vi "log analysis_gps.vi"() -> ()   [LabVIEW 2019] (continued)
0 0\trobot status\t323.592230\t41.689812\t11.246000\t-1.200662\t-1.937489\t150.317707\t0.261000\t0.044000\n\t\n15:30:30.4\tlog_raw\tgps_raw\t\tsystem status\tnormal 2 28.000000 0 0\trobot status\t323.484203\t41.766278\t11.242100\t-1.080469\t-2.157866\t150.215109\t0.275000\t0.023000\n\t\n15:30:30.9\tlog_raw\tgps_raw\t\tsystem status\tnormal 2 28.000000 0 0\trobot status\t323.368044\t41.849297\t11.238300\t-0.983089\t-2.252578\t150.171279\t0.264000\t0.055000\n\t\n15:30:31.4\tlog_raw\tgps_raw\t\tsystem status\tnormal 2 28.000000 0 0\trobot status\t323.251094\t41.933868\t11.233500\t-0.837664\t-2.448431\t150.085808\t0.287000\t0.017000\n\t\n15:30:31.9\tlog_raw\tgps_raw\t#INSPVAXA,USB3,0,50.0,FINESTEERING,2107,282649.900,02000000,471d,15824;INS_ALIGNMENT_COMPLETE,INS_RTKFIXED,37.37050893925,126.72448297158,11.2267,22.3000,0.1903,-0.2023,-0.0241,-0.768669991,-2.369260824,300.015949522,0.4461,0.2933,0.5487,0.1140,0.0923,0.0771,0.0990,0.1039,4.8348,0f000001,0*dea76ac5\n\tsystem status\tnormal 2 28.000000 0 0\trobot status\t323.122038\t42.028367\t11.226700\t-0.768670\t-2.369261\t149.984050\t0.259000\t0.049000\n\t\n15:30:32.4\tlog_raw\tgps_raw\t#INSPVAXA,USB3,0,51.5,FINESTEERING,2107,282650.400,02000000,471d,15824;INS_ALIGNMENT_COMPLETE,INS_RTKFIXED,37.37050972480,126.72448163294,11.2213,22.3000,0.2048,-0.2320,-0.0314,-0.685414349,-2.106294081,300.095837477,0.4453,0.2931,0.5488,0.1140,0.0923,0.0771,0.0990,0.1038,4.8348,0f000001,0*243c57b4\n\tsystem status\tnormal 2 28.000000 0 0\trobot status\t323.003463\t42.115555\t11.221300\t-0.685414\t-2.106294\t149.904163\t0.308000\t-0.015000\n\t\n15:30:32.9\tlog_raw\tgps_raw\t\tsystem status\tnormal 2 28.000000 0 0\trobot status\t322.902785\t42.190545\t11.217300\t-0.695969\t-2.083132\t149.879193\t0.320000\t-0.056000\n\t\n15:30:33.4\tlog_raw\tgps_raw\t\tsystem status\tnormal 2 28.000000 0 0\trobot status\t322.782651\t42.278318\t11.212600\t-0.741534\t-2.009396\t149.782381\t0.332000\t-0.058000\n\t\n15:30:33.9\tlog_raw\tgps_raw\t#INSPVAXA,USB3,0,45.5,FINESTEERING,2107,282651.900,02000000,471d,15824;INS_ALIGNMENT_COMPLETE,INS_RTKFIXED,37.37051201880,126.72447778068,11.2078,22.3000,0.1916,-0.2205,-0.0248,-0.576530745,-1.861777705,300.300269268,0.4449,0.2931,0.5488,0.1139,0.0923,0.0771,0.0990,0.1038,4.8347,0f000001,0*af26017a\n\tsystem status\tnormal 2 28.000000 0 0\trobot status\t322.662236\t42.370167\t11.207800\t-0.576531\t-1.861778\t149.699731\t0.299000\t-0.003000\n\t\n15:30:34.4\tlog_raw\tgps_raw\t\tsystem status\tnormal 2 28.000000 0 0\trobot status\t322.556126\t42.447985\t11.205500\t-0.579348\t-1.879669\t149.599843\t0.304000\t-0.005000\n\t\n15:30:34.9\tlog_raw\tgps_raw\t\tsystem status\tnormal 2 28.000000 0 0\trobot status\t322.440446\t42.533452\t11.202500\t-0.656280\t-1.866283\t149.472784\t0.304000\t-0.004000\n\t\n15:30:35.4\tlog_raw\tgps_raw\t\tsystem status\tnormal 2 28.000000 0 0\trobot status\t322.324996\t42.617118\t11.198800\t-0.815807\t-1.929924\t149.361970\t0.259000\t0.044000\n\t\n15:30:35.9\tlog_raw\tgps_raw\t#INSPVAXA,USB3,0,51.5,FINESTEERING,2107,282653.900,02000000,471d,15824;INS_ALIGNMENT_COMPLETE,INS_RTKFIXED,37.37051509510,126.72447251131,11.1945,22.3000,0.1929,-0.2150,-0.0150,-0.802596336,-1.882184040,300.662762095,0.4446,0.2931,0.5493,0.1139,0.0923,0.0771,0.0991,0.1038,4.8344,0f000001,0*a735d545\n\tsystem status\tnormal 2 28.000000 0 0\trobot status\t322.195484\t42.711607\t11.194500\t-0.802596\t-1.882184\t149.337238\t0.284000\t0.023000\n\t\n15:30:36.4\tlog_raw\tgps_raw\t#INSPVAXA,USB3,0,49.5,FINESTEERING,2107,282654.400,02000000,471d,15824;INS_ALIGNMENT_COMPLETE,INS_RTKFIXED,37.37051584618,126.72447125334,11.1924,22.3000,0.2065,-0.2512,-0.0226,-0.731158373,-1.931164870,300.740729096,0.4441,0.2931,0.5492,0.1141,0.0922,0.0771,0.0991,0.1038,4.8345,0f000001,0*6bec4445\n\tsystem status\tnormal 2 28.000000 0 0\trobot status\t322.084055\t42.794969\t11.192400\t-0.731158\t-1.931165\t149.259271\t0.324000\t-0.010000\n\t\n15:30:36.9\tlog_raw\tgps_raw\t\tsystem status\tnormal 2 28.000000 0 0\trobot status\t321.980427\t42.873038\t11.190300\t-0.706176\t-2.181369\t149.255396\t0.264000\t0.055000\n\t\n15:30:37.4\tlog_raw\tgps_raw\t#INSPVAXA,USB3,0,49.5,FINESTEERING,2107,282655.400,02000000,471d,15824;INS_ALIGNMENT_COMPLETE,INS_RTKFIXED,37.37051739369,126.72446865376,11.1860,22.3000,0.1911,-0.2128,-0.0292,-0.646981835,-2.105939863,300.753498708,0.4442,0.2930,0.5492,0.1138,0.0923,0.0771,0.0991,0.1038,4.8345,0f000001,0*03f7e14e\n\tsystem status\tnormal 2 28.000000 0 0\trobot status\t321.853789\t42.966728\t11.186000\t-0.646982\t-2.105940\t149.246501\t0.252000\t0.069000\n\t\n15:30:37.9\tlog_raw\tgps_raw\t#INSPVAXA,USB3,0,49.5,FINESTEERING,2107,282655.900,02000000,471d,15824;INS_ALIGNMENT_COMPLETE,INS_RTKFIXED,37.37051816950,126.72446734615,11.1828,22.3000,0.1941,-0.2176,-0.0241,-0.579402849,-2.122031776,300.745538986,0.4442,0.2930,0.5492,0.1138,0.0923,0.0771,0.0991,0.1038,4.8345,0f000001,0*dfac7fa4\n\tsystem status\tnormal 2 28.000000 0 0\trobot status\t321.737963\t43.052835\t11.182800\t-0.579403\t-2.122032\t149.254461\t0.290000\t0.030000\n\t\n15:30:38.4\tlog_raw\tgps_raw\t#INSPVAXA,USB3,0,50.0,FINESTEERING,2107,282656.400,02000000,471d,15824;INS_ALIGNMENT_COMPLETE,INS_RTKFIXED,37.37051892940,126.72446603782,11.1784,22.3000,0.1975,-0.2201,-0.0250,-0.527531498,-2.256977557,300.738893590,0.4437,0.2930,0.5489,0.1139,0.0923,0.0771,0.0991,0.1038,4.8347,0f000001,0*858cd015\n\tsystem status\tnormal 2 28.000000 0 0\trobot status\t321.622073\t43.137177\t11.178400\t-0.527531\t-2.256978\t149.261106\t0.264000\t0.075000\n\t\n15:30:38.9\tlog_raw\tgps_raw\t\tsystem status\tnormal 2 28.000000 0 0\trobot status\t321.518741\t43.212547\t11.174000\t-0.494325\t-2.278801\t149.224581\t0.292000\t0.013000\n\t\n15:30:39.4\tlog_raw\tgps_raw\t#INSPVAXA,USB3,0,50.0,FINESTEERING,2107,282657.400,02000000,471d,15824;INS_ALIGNMENT_COMPLETE,INS_RTKFIXED,37.37052044371,126.72446344968,11.1671,22.3000,0.1932,-0.2068,-0.0116,-0.414783465,-2.317412537,300.721707080,0.4433,0.2930,0.5487,0.1138,0.0923,0.0770,0.0992,0.1038,4.8350,0f000001,0*72bd9a4b\n\tsystem status\tnormal 2 28.000000 0 0\trobot status\t321.392820\t43.305251\t11.167100\t-0.414783\t-2.317413\t149.278293\t0.354000\t-0.092000\n\t\n15:30:39.9\tlog_raw\tgps_raw\t#INSPVAXA,USB3,0,50.0,FINESTEERING,2107,282657.900,02000000,471d,15824;INS_ALIGNMENT_COMPLETE,INS_RTKFIXED,37.37052121955,126.72446213298,11.1620,22.3000,0.2017,-0.2233,-0.0206,-0.308273301,-2.524902992,300.688892174,0.4433,0.2930,0.5487,0.1138,0.0923,0.0770,0.0992,0.1038,4.8350,0f000001,0*cf92748e\n\tsystem status\tnormal 2 28.000000 0 0\trobot status\t321.276189\t43.391362\t11.162000\t-0.308273\t-2.524903\t149.311108\t0.298000\t0.014000\n\t\n15:30:40.4\tlog_raw\tgps_raw\t#INSPVAXA,USB3,0,48.0,FINESTEERING,2107,282658.400,02000000,471d,15824;INS_ALIGNMENT_COMPLETE,INS_RTKFIXED,37.37052197544,126.72446081424,11.1558,22.3000,0.2035,-0.2219,-0.0181,-0.328078319,-2.511940655,300.637576073,0.4425,0.2930,0.5482,0.1137,0.0923,0.0770,0.0992,0.1038,4.8355,0f000001,0*376bbad4\n\tsystem status\tnormal 2 28.000000 0 0\trobot status\t321.159377\t43.475258\t11.155800\t-0.328078\t-2.511941\t149.362424\t0.296000\t0.016000\n\t\n15:30:40.9\tlog_raw\tgps_raw\t#INSPVAXA,USB3,0,48.0,FINESTEERING,2107,282658.900,02000000,471d,15824;INS_ALIGNMENT_COMPLETE,INS_RTKFIXED,37.37052272730,126.72445951727,11.1488,22.3000,0.1942,-0.2149,-0.0164,-0.313220820,-2.516289447,300.678904806,0.4425,0.2930,0.5482,0.1137,0.0923,0.0770,0.0992,0.1038,4.8355,0f000001,0*e2928abf\n\tsystem status\tnormal 2 28.000000 0 0\trobot status\t321.044493\t43.558708\t11.148800\t-0.313221\t-2.516289\t149.321095\t0.294000\t0.008000\n\t\n15:30:41.4\tlog_raw\tgps_raw\t\tsystem status\tnormal 2 28.000000 0 0\trobot status\t320.938205\t43.634346\t11.142300\t-0.319450\t-2.549649\t149.279722\t0.273000\t0.030000\n\t\n15:30:41.9\tlog_raw\tgps_raw\t\tsystem status\tnormal 2 28.000000 0 0\trobot status\t320.823860\t43.716526\t11.135800\t-0.322956\t-2.458648\t149.300224\t0.366000\t-0.101000\n\t\n15:30:42.4\tlog_raw\tgps_raw\t#INSPVAXA,USB3,0,50.5,FINESTEERING,2107,282660.400,02000000,471d,15824;INS_ALIGNMENT_COMPLETE,INS_RTKFIXED,37.37052497375,126.72445559407,11.1294,22.3000,0.1977,-0.2195,-0.0225,-0.387313372,-2.271618505,300.730077872,0.4409,0.2929,0.5472,0.1136,0.0922,0.0770,0.0992,0.1038,4.8370,0f000001,0*69452c97\n\tsystem status\tnormal 2 28.000000 0 0\trobot status\t320.696983\t43.808042\t11.129400\t-0.387313\t-2.271619\t149.269922\t0.352000\t-0.076000\n\t\n15:30:42.9\tlog_raw\tgps_raw\t#INSPVAXA,USB3,0,50.5,FINESTEERING,2107,282660.900,02000000,471d,15824;INS_ALIGNMENT_COMPLETE,INS_RTKFIXED,37.37052574047,126.72445427382,11.1237,22.3000,0.1897,-0.2035,-0.0252,-0.381842817,-2.256778592,300.817684769,0.4409,0.2929,0.5472,0.1136,0.0922,0.0770,0.0992,0.1038,4.8370,0f000001,0*d5bdd052\n\tsystem status\tnormal 2 28.000000 0 0\trobot status\t320.580037\t43.893141\t11.123700\t-0.381843\t-2.256779\t149.182315\t0.278000\t0.020000\n\t\n15:30:43.4\tlog_raw\tgps_raw\t#INSPVAXA,USB3,0,49.5,FINESTEERING,2107,282661.400,02000000,471d,15824;INS_ALIGNMENT_COMPLETE,INS_RTKFIXED,37.37052651141,126.72445295109,11.1180,22.3000,0.1959,-0.2165,-0.0224,-0.305806610,-2.215640419,300.881180775,0.4410,0.2930,0.5471,0.1137,0.0922,0.0770,0.0993,0.1038,4.8381,0f000001,0*01198745\n\tsystem status\tnormal 2 28.000000 0 0\trobot status\t320.462872\t43.978708\t11.118000\t-0.305807\t-2.215640\t149.118819\t0.281000\t0.027000\n\t\n15:30:43.9\tlog_raw\tgps_raw\t#INSPVAXA,USB3,0,49.5,FINESTEERING,2107,282661.900,02000000,471d,15824;INS_ALIGNMENT_COMPLETE,INS_RTKFIXED,37.37052725992,126.72445165392,11.1131,22.3000,0.1958,-0.2218,-0.0300,-0.421587704,-2.162878960,300.913228762,0.4410,0.2930,0.5471,0.1137,0.0922,0.0770,0.0993,0.1038,4.8381,0f000001,0*8e192d49\n\tsystem status\tnormal 2 28.000000 0 0\trobot status\t320.347971\t44.061785\t11.113100\t-0.421588\t-2.162879\t149.086771\t0.249000\t0.076000\n\t\n15:30:44.4\tlog_raw\tgps_raw\t#INSPVAXA,USB3,0,52.0,FINESTEERING,2107,282662.400,02000000,471d,15824;INS_ALIGNMENT_COMPLETE,INS_RTKFIXED,37.37052801675,126.72445034380,11.1087,22.3000,0.1896,-0.2102,-0.0176,-0.535002925,-2.143447457,300.990757797,0.4412,0.2930,0.5470,0.1137,0.0922,0.0770,0.0993,0.1038,4.8391,0f000001,0*8c4251fb\n\tsystem status\tnormal 2 28.000000 0 0\trobot status\t320.231923\t44.145786\t11.108700\t-0.535003\t-2.143447\t149.009242\t0.338000\t-0.068000\n\t\n15:30:44.9\tlog_raw\tgps_raw\t#INSPVAXA,USB3,0,52.0,FINESTEERING,2107,282662.900,02000000,471d,15824;INS_ALIGNMENT_COMPLETE,INS_RTKFIXED,37.37052880342,126.72444898642,11.1040,22.3000,0.1905,-0.2142,-0.0217,-0.575840592,-2.161837706,301.070112972,0.4412,0.2930,0.5470,0.1137,0.0922,0.0770,0.0993,0.1038,4.8391,0f000001,0*2ee126c6\n\tsystem status\tnormal 2 28.000000 0 0\trobot status\t320.111688\t44.233099\t11.104000\t-0.575841\t-2.161838\t148.929887\t0.338000\t-0.057000\n\t\n15:30:45.4\tlog_raw\tgps_raw\t#INSPVAXA,USB3,0,49.0,FINESTEERING,2107,282663.400,02000000,471d,15824;INS_ALIGNMENT_COMPLETE,INS_RTKFIXED,37.37052954535,126.72444770805,11.0993,22.3000,0.2098,-0.2404,-0.0214,-0.590246803,-1.901325753,301.153923627,0.4417,0.2932,0.5470,0.1139,0.0924,0.0770,0.0993,0.1038,4.8402,0f000001,0*c89c711f\n\tsystem status\tnormal 2 28.000000 0 0\trobot status\t319.998452\t44.315446\t11.099300\t-0.590247\t-1.901326\t148.846076\t0.316000\t-0.007000\n\t\n15:30:45.9\tlog_raw\tgps_raw\t#DUALANTENNAHEADINGA,USB3,0,49.0,FINESTEERING,2107,282663.900,02000000,d426,15824;SOL_COMPUTED,L1_FLOAT,-1.000000000,333.457733154,12.245697021,0.0,360.000000000,180.000000000,\"631T\",15,5,5,5,04,00,20,20*8b83e92e\n\tsystem status\tnormal 2 28.000000 0 0\trobot status\t319.882796\t44.400006\t11.094000\t-0.573003\t-1.990010\t148.718791\t0.281000\t0.026000\n\t\n15:30:46.4\tlog_raw\tgps_raw\t#INSPVAXA,USB3,0,45.5,FINESTEERING,2107,282664.400,02000000,471d,15824;INS_ALIGNMENT_COMPLETE,INS_RTKFIXED,37.37053109061,126.72444506207,11.0879,22.3000,0.1993,-0.2262,-0.0239,-0.578200163,-2.123585690,301.384652379,0.4420,0.2933,0.5470,0.1138,0.0924,0.0770,0.0993,0.1038,4.8409,0f000001,0*2eda5995\n\tsystem status\tnormal 2 28.000000 0 0\trobot status\t319.764076\t44.486955\t11.087900\t-0.578200\t-2.123586\t148.615348\t0.301000\t-0.011000\n\t\n15:30:46.9\tlog_raw\tgps_raw\t#INSPVAXA,USB3,0,45.5,FINESTEERING,2107,282664.900,02000000,471d,15824;INS_ALIGNMENT_COMPLETE,INS_RTKFIXED,37.37053183209,126.72444381821,11.0830,22.3000,0.2025,-0.2395,-0.0183,-0.627563942,-2.176125382,301.462972604,0.4420,0.2933,0.5470,0.1138,0.0924,0.0770,0.0993,0.1038,4.8409,0f000001,0*51325076\n\tsystem status\tnormal 2 28.000000 0 0\trobot status\t319.653896\t44.569253\t11.083000\t-0.627564\t-2.176125\t148.537027\t0.317000\t-0.016000\n\t\n15:30:47.4\tlog_raw\tgps_raw\t#INSPVAXA,USB3,0,50.5,FINESTEERING,2107,282665.400,02000000,471d,15824;INS_ALIGNMENT_COMPLETE,INS_RTKFIXED,37.37053260836,126.72444247630,11.0777,22.3000,0.1697,-0.2000,-0.0233,-0.806380731,-2.428315608,301.586666898,0.4420,0.2935,0.5472,0.1137,0.0923,0.0770,0.0992,0.1038,4.8415,0f000001,0*d8a31360\n\tsystem status\tnormal 2 28.000000 0 0\trobot status\t319.535032\t44.655411\t11.077700\t-0.806381\t-2.428316\t148.413333\t0.343000\t-0.075000\n\t\n15:30:47.9\tlog_raw\tgps_raw\t#INSPVAXA,USB3,0,50.5,FINESTEERING,2107,282665.900,02000000,471d,15824;INS_ALIGNMENT_COMPLETE,INS_RTKFIXED,37.37053337130,126.72444116871,11.0726,22.3000,0.1954,-0.2209,-0.0080,-0.903161753,-2.476998563,301.699215129,0.4420,0.2935,0.5472,0.1137,0.0923,0.0770,0.0992,0.1038,4.8415,0f000001,0*b607e80f\n\tsystem status\tnormal 2 28.000000 0 0\trobot status\t319.419208\t44.740090\t11.072600\t-0.903162\t-2.476999\t148.300785\t0.302000\t-0.002000\n\t\n15:30:48.4\tlog_raw\tgps_raw\t#DUALANTENNAHEADINGA,USB3,0,47.0,FINESTEERING,2107,282666.400,02000000,d426,15824;INSUFFICIENT_OBS,NONE,-1.000000000,0.000000000,0.000000000,0.0,0.000000000,0.000000000,\"631T\",14,3,3,3,04,00,20,00*a6710081\n\tsystem status\tnormal 2 28.000000 0 0\trobot status\t319.307124\t44.820469\t11.065800\t-0.991680\t-2.437730\t148.216492\t0.350000\t-0.079000\n\t\n15:30:48.9\tlog_raw\tgps_raw\t#INSPVAXA,USB3,0,47.0,FINESTEERING,2107,282666.900,02000000,471d,15824;INS_ALIGNMENT_COMPLETE,INS_RTKFIXED,37.37053484048,126.72443859916,11.0582,22.3000,0.1830,-0.2119,-0.0311,-0.968807751,-2.464707022,301.855553753,0.4415,0.2935,0.5473,0.1137,0.0925,0.0771,0.0992,0.1038,4.8423,0f000001,0*59f4e239\n\tsystem status\tnormal 2 28.000000 0 0\trobot status\t319.191602\t44.903155\t11.058200\t-0.968808\t-2.464707\t148.144446\t0.254000\t0.066000\n\t\n15:30:49.4\tlog_raw\tgps_raw\t#DUALANTENNAHEADINGA,USB3,0,49.5,FINESTEERING,2107,282667.400,02000000,d426,15824;INSUFFICIENT_OBS,NONE,-1.000000000,0.000000000,0.000000000,0.0,0.000000000,0.000000000,\"631T\",15,3,3,3,04,00,20,00*5f1e2af7\n\tsystem status\tnormal 2 28.000000 0 0\trobot status\t319.076990\t44.987112\t11.050700\t-0.932653\t-2.446780\t148.027848\t0.283000\t0.017000\n\t\n15:30:49.9\tlog_raw\tgps_raw\t#INSPVAXA,USB3,0,49.5,FINESTEERING,2107,282667.900,02000000,471d,15824;INS_ALIGNMENT_COMPLETE,INS_RTKFIXED,37.37053633502,126.72443604770,11.0435,22.3000,0.1822,-0.2080,-0.0221,-0.962443537,-2.273211285,302.003209651,0.4405,0.2936,0.5472,0.1136,0.0924,0.0770,0.0991,0.1038,4.8429,0f000001,0*2d8cca71\n\tsystem status\tnormal 2 28.000000 0 0\trobot status\t318.965597\t45.069035\t11.043500\t-0.962444\t-2.273211\t147.996790\t0.256000\t0.047000\n\t\n15:30:50.4\tlog_raw\tgps_raw\t#DUALANTENNAHEADINGA,USB3,0,51.0,FINESTEERING,2107,282668.400,02000000,d426,15824;INSUFFICIENT_OBS,NONE,-1.000000000,0.000000000,0.000000000,0.0,0.000000000,0.000000000,\"631T\",13,3,3,3,04,00,20,00*d0f86fa9\n\tsystem status\tnormal 2 28.000000 0 0\trobot status\t318.849663\t45.153830\t11.037600\t-0.906958\t-2.251266\t147.906324\t0.279000\t0.013000\n\t\n15:30:50.9\tlog_raw\tgps_raw\t#INSPVAXA,USB3,0,51.0,FINESTEERING,2107,282668.900,02000000,471d,15824;INS_ALIGNMENT_COMPLETE,INS_RTKFIXED,37.37053784422,126.72443343900,11.0314,22.3000,0.1770,-0.2175,-0.0238,-1.067658542,-2.117354473,302.168245726,0.4406,0.2938,0.5474,0.1136,0.0926,0.0771,0.0991,0.1038,4.8433,0f000001,0*743eb533\n\tsystem status\tnormal 2 28.000000 0 0\trobot status\t318.734523\t45.236541\t11.031400\t-1.067659\t-2.117354\t147.831754\t0.290000\t0.007000\n\t\n15:30:51.4\tlog_raw\tgps_raw\t#INSPVAXA,USB3,0,50.5,FINESTEERING,2107,282669.400,02000000,471d,15824;INS_ALIGNMENT_COMPLETE,INS_RTKFIXED,37.37053859261,126.72443216227,11.0246,22.3000,0.1748,-0.2150,-0.0262,-1.134800808,-1.987218323,302.206484559,0.4410,0.2939,0.5476,0.1137,0.0929,0.0771,0.0990,0.1039,4.8430,0f000001,0*0ef77350\n\tsystem status\tnormal 2 28.000000 0 0\trobot status\t318.621432\t45.319606\t11.024600\t-1.134801\t-1.987218\t147.793515\t0.292000\t0.005000\n\t\n15:30:51.9\tlog_raw\tgps_raw\t#INSPVAXA,USB3,0,50.5,FINESTEERING,2107,282669.900,02000000,471d,15824;INS_ALIGNMENT_COMPLETE,INS_RTKFIXED,37.37053936070,126.72443086861,11.0170,22.3000,0.1679,-0.2152,-0.0201,-1.047863329,-2.047137616,302.259088217,0.4410,0.2939,0.5476,0.1137,0.0929,0.0771,0.0990,0.1039,4.8430,0f000001,0*b3a345e1\n\tsystem status\tnormal 2 28.000000 0 0\trobot status\t318.506842\t45.404856\t11.017000\t-1.047863\t-2.047138\t147.740912\t0.279000\t0.012000\n\t\n15:30:52.4\tlog_raw\tgps_raw\t#INSPVAXA,USB3,0,51.5,FINESTEERING,2107,282670.400,02000000,471d,15824;INS_ALIGNMENT_COMPLETE,INS_RTKFIXED,37.37054013304,126.72442955163,11.0107,22.3000,0.1797,-0.2154,-0.0330,-1.008775367,-2.075430336,302.292083469,0.4412,0.2940,0.5477,0.1137,0.0927,0.0771,0.0989,0.1039,4.8414,0f000001,0*6124701b\n\tsystem status\tnormal 2 28.000000 0 0\trobot status\t318.390186\t45.490578\t11.010700\t-1.008775\t-2.075430\t147.707917\t0.281000\t0.028000\n\t\n15:30:52.9\tlog_raw\tgps_raw\t#INSPVAXA,USB3,0,51.5,FINESTEERING,2107,282670.900,02000000,471d,15824;INS_ALIGNMENT_COMPLETE,INS_RTKFIXED,37.37054088934,126.72442826376,11.0051,22.3000,0.1741,-0.2301,-0.0351,-1.043464274,-1.977986056,302.323016199,0.4412,0.2940,0.5477,0.1137,0.0927,0.0771,0.0989,0.1039,4.8414,0f000001,0*5cd64784\n\tsystem status\tnormal 2 28.000000 0 0\trobot status\t318.276109\t45.574520\t11.005100\t-1.043464\t-1.977986\t147.676984\t0.264000\t0.057000\n\t\n15:30:53.4\tlog_raw\tgps_raw\t#INSPVAXA,USB3,0,51.0,FINESTEERING,2107,282671.400,02000000,471d,15824;INS_ALIGNMENT_COMPLETE,INS_RTKFIXED,37.37054164500,126.72442698236,10.9999,22.3000,0.1651,-0.2207,-0.0264,-1.152870335,-2.003288963,302.368323626,0.4421,0.2942,0.5481,0.1138,0.0926,0.0771,0.0989,0.1039,4.8395,0f000001,0*729e65cc\n\tsystem status\tnormal 2 28.000000 0 0\trobot status\t318.162604\t45.658391\t10.999900\t-1.152870\t-2.003289\t147.631676\t0.280000\t0.012000\n\t\n15:30:53.9\tlog_raw\tgps_raw\t#DUALANTENNAHEADINGA,USB3,0,51.0,FINESTEERING,2107,282671.900,02000000,d426,15824;SOL_COMPUTED,L1_FLOAT,-1.000000000,6.424537182,-37.266357422,0.0,360.000000000,180.000000000,\"631T\",14,5,5,5,04,00,20,20*1315aa76\n\tsystem status\tnormal 2 28.000000 0 0\trobot status\t318.046362\t45.744272\t10.995100\t-1.228635\t-2.007328\t147.603662\t0.372000\t-0.119000\n\t\n15:30:54.4\tlog_raw\tgps_raw\t#INSPVAXA,USB3,0,52.5,FINESTEERING,2107,282672.400,02000000,471d,15824;INS_ALIGNMENT_COMPLETE,INS_RTKFIXED,37.37054317479,126.72442436870,10.9904,22.3000,0.1725,-0.2321,-0.0318,-1.253314249,-1.912910767,302.408086274,0.4431,0.2945,0.5488,0.1140,0.0927,0.0771,0.0988,0.1039,4.8375,0f000001,0*4ca87b98\n\tsystem status\tnormal 2 28.000000 0 0\trobot status\t317.931091\t45.828183\t10.990400\t-1.253314\t-1.912911\t147.591914\t0.369000\t-0.099000\n\t\n15:30:54.9\tlog_raw\tgps_raw\t#INSPVAXA,USB3,0,52.5,FINESTEERING,2107,282672.900,02000000,471d,15824;INS_ALIGNMENT_COMPLETE,INS_RTKFIXED,37.37054392116,126.72442309351,10.9862,22.3000,0.1660,-0.2327,-0.0240,-1.192361701,-1.928177514,302.476152160,0.4431,0.2945,0.5488,0.1140,0.0927,0.0771,0.0988,0.1039,4.8375,0f000001,0*83cc3094\n\tsystem status\tnormal 2 28.000000 0 0\trobot status\t317.818136\t45.911023\t10.986200\t-1.192362\t-1.928178\t147.523848\t0.345000\t-0.069000\n\t\n15:30:55.4\tlog_raw\tgps_raw\t#INSPVAXA,USB3,0,51.5,FINESTEERING,2107,282673.400,02000000,471d,15824;INS_ALIGNMENT_COMPLETE,INS_RTKFIXED,37.37054468191,126.72442179361,10.9818,22.3000,0.1549,-0.2194,-0.0237,-1.138544711,-1.857754611,302.526216112,0.4445,0.2949,0.5496,0.1141,0.0925,0.0772,0.0988,0.1040,4.8352,0f000001,0*601d5af9\n\tsystem status\tnormal 2 28.000000 0 0\trobot status\t317.702993\t45.995459\t10.981800\t-1.138545\t-1.857755\t147.473784\t0.245000\t0.064000\n\t\n15:30:55.9\tlog_raw\tgps_raw\t#INSPVAXA,USB3,0,51.5,FINESTEERING,2107,282673.900,02000000,471d,15824;INS_ALIGNMENT_COMPLETE,INS_RTKFIXED,37.37054544133,126.72442048455,10.9776,22.3000,0.1608,-0.2204,-0.0208,-1.194325383,-1.773338448,302.575514269,0.4445,0.2949,0.5496,0.1141,0.0925,0.0772,0.0988,0.1040,4.8352,0f000001,0*3c4b28bd\n\tsystem status\tnormal 2 28.000000 0 0\trobot status\t317.587039\t46.079747\t10.977600\t-1.194325\t-1.773338\t147.424486\t0.245000\t0.076000\n\t\n15:30:56.4\tlog_raw\tgps_raw\t#DUALANTENNAHEADINGA,USB3,0,52.0,FINESTEERING,2107,282674.400,02000000,d426,15824;INSUFFICIENT_OBS,NONE,-1.000000000,0.000000000,0.000000000,0.0,0.000000000,0.000000000,\"631T\",11,3,3,3,04,00,20,00*43d09faf\n\tsystem status\tnormal 2 28.000000 0 0\trobot status\t317.471513\t46.163234\t10.972700\t-1.309159\t-1.774480\t147.324910\t0.285000\t0.020000\n\t\n15:30:56.9\tlog_raw\tgps_raw\t#INSPVAXA,USB3,0,52.0,FINESTEERING,2107,282674.900,02000000,471d,15824;INS_ALIGNMENT_COMPLETE,INS_RTKFIXED,37.37054694617,126.72441789266,10.9675,22.3000,0.1711,-0.2297,-0.0188,-1.275138168,-1.781517765,302.710392132,0.4449,0.2948,0.5501,0.1143,0.0927,0.0772,0.0987,0.1040,4.8338,0f000001,0*704fcea3\n\tsystem status\tnormal 2 28.000000 0 0\trobot status\t317.357454\t46.246770\t10.967500\t-1.275138\t-1.781518\t147.289608\t0.262000\t0.043000\n\t\n15:30:57.4\tlog_raw\tgps_raw\t#INSPVAXA,USB3,0,50.5,FINESTEERING,2107,282675.400,02000000,471d,15824;INS_ALIGNMENT_COMPLETE,INS_RTKFIXED,37.37054775333,126.72441659154,10.9642,22.3000,0.1645,-0.2327,-0.0094,-1.051395479,-1.879417233,302.757545593,0.4453,0.2948,0.5504,0.1142,0.0925,0.0772,0.0987,0.1040,4.8321,0f000001,0*a4c6f5d9\n\tsystem status\tnormal 2 28.000000 0 0\trobot status\t317.242203\t46.336357\t10.964200\t-1.051395\t-1.879417\t147.242454\t0.279000\t0.028000\n\t\n15:30:57.9\tlog_raw\tgps_raw\t#DUALANTENNAHEADINGA,USB3,0,50.5,FINESTEERING,2107,282675.900,02000000,d426,15824;INSUFFICIENT_OBS,NONE,-1.000000000,0.000000000,0.000000000,0.0,0.000000000,0.000000000,\"631T\",14,3,3,3,04,00,20,00*348e632d\n\tsystem status\tnormal 2 28.000000 0 0\trobot status\t317.128394\t46.425056\t10.962400\t-1.001695\t-1.938068\t147.172173\t0.263000\t0.060000\n\t\n15:30:58.4\tlog_raw\tgps_raw\t#INSPVAXA,USB3,0,48.5,FINESTEERING,2107,282676.400,02000000,471d,15824;INS_ALIGNMENT_COMPLETE,INS_RTKFIXED,37.37054934080,126.72441402594,10.9604,22.3000,0.1664,-0.2342,-0.0147,-1.030303751,-1.986468861,302.910679697,0.4460,0.2946,0.5508,0.1143,0.0923,0.0772,0.0987,0.1040,4.8310,0f000001,0*713be666\n\tsystem status\tnormal 2 28.000000 0 0\trobot status\t317.014946\t46.512550\t10.960400\t-1.030304\t-1.986469\t147.089320\t0.346000\t-0.074000\n\t\n15:30:58.9\tlog_raw\tgps_raw\t#INSPVAXA,USB3,0,48.5,FINESTEERING,2107,282676.900,02000000,471d,15824;INS_ALIGNMENT_COMPLETE,INS_RTKFIXED,37.37055013334,126.72441273552,10.9584,22.3000,0.1604,-0.2244,-0.0102,-1.040479369,-1.905860693,302.964821011,0.4460,0.2946,0.5508,0.1143,0.0923,0.0772,0.0987,0.1040,4.8310,0f000001,0*b8bc8b15\n\tsystem status\tnormal 2 28.000000 0 0\trobot status\t316.900643\t46.600514\t10.958400\t-1.040479\t-1.905861\t147.035179\t0.340000\t-0.069000\n\t\n15:30:59.4\tlog_raw\tgps_raw\t#INSPVAXA,USB3,0,50.5,FINESTEERING,2107,282677.400,02000000,471d,15824;INS_ALIGNMENT_COMPLETE,INS_RTKFIXED,37.37055094880,126.72441141455,10.9545,22.3000,0.1625,-0.2172,-0.0160,-0.890769170,-1.829812831,303.004445292,0.4467,0.2944,0.5513,0.1144,0.0924,0.0772,0.0987,0.1040,4.8309,0f000001,0*53662f9b\n\tsystem status\tnormal 2 28.000000 0 0\trobot status\t316.783633\t46.691022\t10.954500\t-0.890769\t-1.829813\t146.995555\t0.287000\t0.016000\n\t\n15:30:59.9\tlog_raw\tgps_raw\t#DUALANTENNAHEADINGA,USB3,0,50.5,FINESTEERING,2107,282677.900,02000000,d426,15824;INSUFFICIENT_OBS,NONE,-1.000000000,0.000000000,0.000000000,0.0,0.000000000,0.000000000,\"631T\",15,3,3,3,04,00,20,00*38dceac7\n\tsystem status\tnormal 2 28.000000 0 0\trobot status\t316.669015\t46.779335\t10.950600\t-0.841043\t-1.839368\t146.965521\t0.289000\t0.017000\n\t\n15:31:00.4\tlog_raw\tgps_raw\t#INSPVAXA,USB3,0,43.0,FINESTEERING,2107,282678.400,02000000,471d,15824;INS_ALIGNMENT_COMPLETE,INS_RTKFIXED,37.37055255572,126.72440886198,10.9468,22.3000,0.1687,-0.2243,-0.0108,-0.678924233,-1.833067267,303.044860891,0.4469,0.2942,0.5516,0.1145,0.0924,0.0772,0.0987,0.1040,4.8313,0f000001,0*bb99175a\n\tsystem status\tnormal 2 28.000000 0 0\trobot status\t316.557531\t46.869374\t10.946800\t-0.678924\t-1.833067\t146.955139\t0.280000\t0.028000\n\t\n15:31:00.9\tlog_raw\tgps_raw\t#DUALANTENNAHEADINGA,USB3,0,43.0,FINESTEERING,2107,282678.900,02000000,d426,15824;INSUFFICIENT_OBS,NONE,-1.000000000,0.000000000,0.000000000,0.0,0.000000000,0.000000000,\"631T\",14,3,3,3,04,00,20,00*c50de69c\n\tsystem status\tnormal 2 28.000000 0 0\trobot status\t316.442410\t46.961952\t10.941700\t-0.614706\t-2.092216\t146.922740\t0.284000\t0.021000\n\t\n15:31:01.4\tlog_raw\tgps_raw\t#DUALANTENNAHEADINGA,USB3,0,51.0,FINESTEERING,2107,282679.400,02000000,d426,15824;SOL_COMPUTED,L1_FLOAT,-1.000000000,21.335779190,-47.169494629,0.0,193.181869507,129.996200562,\"631T\",14,5,5,5,04,00,20,20*2871a391\n\tsystem status\tnormal 2 28.000000 0 0\trobot status\t316.326513\t47.054096\t10.936900\t-0.664086\t-2.266432\t146.929159\t0.294000\t0.015000\n\t\n15:31:01.9\tlog_raw\tgps_raw\t#DUALANTENNAHEADINGA,USB3,0,51.0,FINESTEERING,2107,282679.900,02000000,d426,15824;SOL_COMPUTED,L1_FLOAT,-1.000000000,20.963815689,-49.860382080,0.0,193.921173096,108.310935974,\"631T\",14,5,5,5,04,00,20,20*13dab214\n\tsystem status\tnormal 2 28.000000 0 0\trobot status\t316.214951\t47.142936\t10.932200\t-0.738157\t-2.215484\t146.944908\t0.378000\t-0.110000\n\t\n15:31:02.4\tlog_raw\tgps_raw\t#INSPVAXA,USB3,0,49.5,FINESTEERING,2107,282680.400,02000000,471d,15824;INS_ALIGNMENT_COMPLETE,INS_RTKFIXED,37.37055584590,126.72440372212,10.9267,22.3000,0.1683,-0.2234,-0.0175,-0.724680252,-2.288934243,303.019606078,0.4465,0.2938,0.5517,0.1142,0.0925,0.0772,0.0987,0.1039,4.8325,0f000001,0*ef175975\n\tsystem status\tnormal 2 28.000000 0 0\trobot status\t316.102250\t47.234551\t10.926700\t-0.724680\t-2.288934\t146.980394\t0.363000\t-0.107000\n\t\n15:31:02.9\tlog_raw\tgps_raw\t#DUALANTENNAHEADINGA,USB3,0,49.5,FINESTEERING,2107,282680.900,02000000,d426,15824;SOL_COMPUTED,L1_FLOAT,-1.000000000,17.254264832,-46.720001221,0.0,249.251464844,160.460342407,\"631T\",15,5,5,5,04,00,20,20*4935c559\n\tsystem status\tnormal 2 28.000000 0 0\trobot status\t315.989276\t47.327762\t10.920800\t-0.643846\t-2.291059\t146.971712\t0.293000\t0.016000\n\t\n15:31:03.4\tlog_raw\tgps_raw\t#DUALANTENNAHEADINGA,USB3,0,52.0,FINESTEERING,2107,282681.400,02000000,d426,15824;SOL_COMPUTED,L1_FLOAT,-1.000000000,5.197163105,-35.837677002,0.0,360.000000000,180.000000000,\"631T\",15,5,5,5,04,00,20,20*e552e6d0\n\tsystem status\tnormal 2 28.000000 0 0\trobot status\t315.879348\t47.417928\t10.915100\t-0.610806\t-2.088467\t146.990071\t0.265000\t0.066000\n\t\n15:31:03.9\tlog_raw\tgps_raw\t#DUALANTENNAHEADINGA,USB3,0,52.0,FINESTEERING,2107,282681.900,02000000,d426,15824;SOL_COMPUTED,L1_FLOAT,-1.000000000,5.226606846,-33.722320557,0.0,360.000000000,180.000000000,\"631T\",14,5,5,5,04,00,20,20*81528f45\n\tsystem status\tnormal 2 28.000000 0 0\trobot status\t315.770203\t47.506372\t10.910300\t-0.674928\t-1.971996\t147.020191\t0.382000\t-0.110000\n\t\n15:31:04.4\tlog_raw\tgps_raw\t#DUALANTENNAHEADINGA,USB3,0,46.5,FINESTEERING,2107,282682.400,02000000,d426,15824;SOL_COMPUTED,L1_FLOAT,-1.000000000,356.926879883,-21.442382813,0.0,360.000000000,180.000000000,\"631T\",14,5,5,5,04,00,20,20*df144227\n\tsystem status\tnormal 2 28.000000 0 0\trobot status\t315.658205\t47.596569\t10.904400\t-0.646854\t-1.943235\t147.093245\t0.264000\t0.042000\n\t\n15:31:04.9\tlog_raw\tgps_raw\t#DUALANTENNAHEADINGA,USB3,0,46.5,FINESTEERING,2107,282682.900,02000000,d426,15824;SOL_COMPUTED,L1_FLOAT,-1.000000000,355.913299561,-34.093353271,0.0,360.000000000,180.000000000,\"631T\",16,5,5,5,04,00,20,20*8a484d88\n\tsystem status\tnormal 2 28.000000 0 0\trobot status\t315.545824\t47.685906\t10.898200\t-0.703628\t-1.913974\t147.170923\t0.319000\t-0.026000\n\t\n15:31:05.4\tlog_raw\tgps_raw\t#INSPVAXA,USB3,0,47.5,FINESTEERING,2107,282683.400,02008000,471d,15824;INS_ALIGNMENT_COMPLETE,INS_RTKFIXED,37.37056070988,126.72439621643,10.8934,22.3000,0.1823,-0.2154,-0.0338,-0.633682870,-1.700441469,302.701865848,0.4459,0.2937,0.5514,0.1144,0.0924,0.0772,0.0987,0.1039,4.8335,0f000001,0*fab402d9\n\tsystem status\tnormal 2 28.000000 0 0\trobot status\t315.437409\t47.774403\t10.893400\t-0.633683\t-1.700441\t147.298134\t0.283000\t0.034000\n\t\n15:31:05.9\tlog_raw\tgps_raw\t#INSPVAXA,USB3,0,47.5,FINESTEERING,2107,282683.900,02008000,471d,15824;INS_ALIGNMENT_COMPLETE,INS_RTKFIXED,37.37056151412,126.72439497192,10.8876,22.3000,0.1856,-0.2259,-0.0357,-0.593256165,-1.575198052,302.563875130,0.4459,0.2937,0.5514,0.1144,0.0924,0.0772,0.0987,0.1039,4.8335,0f000001,0*6eaca9c0\n\tsystem status\tnormal 2 28.000000 0 0\trobot status\t315.327172\t47.863665\t10.887600\t-0.593256\t-1.575198\t147.436125\t0.302000\t0.005000\n\t\n15:31:06.4\tlog_raw\tgps_raw\t#DUALANTENNAHEADINGA,USB3,0,48.0,FINESTEERING,2107,282684.400,02008000,d426,15824;INSUFFICIENT_OBS,NONE,-1.000000000,0.000000000,0.000000000,0.0,0.000000000,0.000000000,\"631T\",14,3,3,3,04,00,20,00*e1343e52\n\tsystem status\tnormal 2 28.000000 0 0\trobot status\t315.215817\t47.954627\t10.882200\t-0.523758\t-1.453583\t147.542580\t0.240000\t0.093000\n\t\n15:31:06.9\tlog_raw\tgps_raw\t#DUALANTENNAHEADINGA,USB3,0,48.0,FINESTEERING,2107,282684.900,02008000,d426,15824;INSUFFICIENT_OBS,NONE,-1.000000000,0.000000000,0.000000000,0.0,0.000000000,0.000000000,\"631T\",14,3,3,3,04,00,20,00*58cb0037\n\tsystem status\tnormal 2 28.000000 0 0\trobot status\t315.105468\t48.045002\t10.877600\t-0.542812\t-1.470202\t147.681333\t0.338000\t-0.060000\n\t\n15:31:07.4\tlog_raw\tgps_raw\t#DUALANTENNAHEADINGA,USB3,0,50.0,FINESTEERING,2107,282685.400,02008000,d426,15824;INSUFFICIENT_OBS,NONE,-1.000000000,0.000000000,0.000000000,0.0,0.000000000,0.000000000,\"631T\",15,3,3,3,04,00,20,00*1e152056\n\tsystem status\tnormal 2 28.000000 0 0\trobot status\t314.996527\t48.133490\t10.873900\t-0.550222\t-1.343344\t147.836850\t0.255000\t0.069000\n\t\n15:31:07.9\tlog_raw\tgps_raw\t#DUALANTENNAHEADINGA,USB3,0,50.0,FINESTEERING,2107,282685.900,02008000,d426,15824;INSUFFICIENT_OBS,NONE,-1.000000000,0.000000000,0.000000000,0.0,0.000000000,0.000000000,\"631T\",15,3,3,3,04,00,20,00*a7ea1e33\n\tsystem status\tnormal 2 28.000000 0 0\trobot status\t314.884282\t48.224876\t10.870300\t-0.458197\t-1.593538\t148.001483\t0.267000\t0.061000\n\t\n15:31:08.4\tlog_raw\tgps_raw\t#INSPVAXA,USB3,0,47.0,FINESTEERING,2107,282686.400,02008000,471d,15824;INS_ALIGNMENT_COMPLETE,INS_RTKFIXED,37.37056557594,126.72438871297,10.8671,22.3000,0.1902,-0.2071,-0.0220,-0.466180041,-1.620819685,301.862974006,0.4463,0.2937,0.5510,0.1145,0.0924,0.0772,0.0987,0.1039,4.8334,0f000001,0*000637b1\n\tsystem status\tnormal 2 27.900000 0 0\trobot status\t314.772765\t48.314485\t10.867100\t-0.466180\t-1.620820\t148.137026\t0.346000\t-0.048000\n\t\n15:31:08.9\tlog_raw\tgps_raw\t#DUALANTENNAHEADINGA,USB3,0,47.0,FINESTEERING,2107,282686.900,02008000,d426,15824;INSUFFICIENT_OBS,NONE,-1.000000000,0.000000000,0.000000000,0.0,0.000000000,0.000000000,\"631T\",15,3,3,3,04,00,20,00*26f21742\n\tsystem status\tnormal 2 28.000000 0 0\trobot status\t314.663718\t48.402728\t10.863600\t-0.392370\t-1.597483\t148.342549\t0.253000\t0.071000\n\t\n15:31:09.4\tlog_raw\tgps_raw\t#DUALANTENNAHEADINGA,USB3,0,48.0,FINESTEERING,2107,282687.400,02000000,d426,15824;INSUFFICIENT_OBS,NONE,-1.000000000,0.000000000,0.000000000,0.0,0.000000000,0.000000000,\"631T\",15,3,3,3,04,00,20,00*962d37c0\n\tsystem status\tnormal 2 28.000000 0 0\trobot status\t314.552017\t48.490482\t10.859200\t-0.302538\t-1.790898\t148.518451\t0.327000\t-0.040000\n\t\n15:31:09.9\tlog_raw\tgps_raw\t#INSPVAXA,USB3,0,48.0,FINESTEERING,2107,282687.900,02000000,471d,15824;INS_ALIGNMENT_COMPLETE,INS_RTKFIXED,37.37056796292,126.72438494002,10.8533,22.3000,0.1859,-0.2072,-0.0348,-0.193858234,-1.879869364,301.375328735,0.4457,0.2937,0.5507,0.1142,0.0925,0.0771,0.0987,0.1038,4.8329,0f000001,0*d3beefd5\n\tsystem status\tnormal 2 28.000000 0 0\trobot status\t314.438563\t48.579416\t10.853300\t-0.193858\t-1.879869\t148.624671\t0.338000\t-0.061000\n\t\n15:31:10.4\tlog_raw\tgps_raw\t#DUALANTENNAHEADINGA,USB3,0,47.0,FINESTEERING,2107,282688.400,02000000,d426,15824;INSUFFICIENT_OBS,NONE,-1.000000000,0.000000000,0.000000000,0.0,0.000000000,0.000000000,\"631T\",13,3,3,3,04,00,20,00*7bc19048\n\tsystem status\tnormal 2 27.900000 0 0\trobot status\t314.324756\t48.666801\t10.846900\t-0.115688\t-2.058051\t148.801968\t0.343000\t-0.076000\n\t\n15:31:10.9\tlog_raw\tgps_raw\t#DUALANTENNAHEADINGA,USB3,0,47.0,FINESTEERING,2107,282688.900,02000000,d426,15824;INSUFFICIENT_OBS,NONE,-1.000000000,0.000000000,0.000000000,0.0,0.000000000,0.000000000,\"631T\",16,3,3,3,04,00,20,00*fcb42397\n\tsystem status\tnormal 2 27.900000 0 0\trobot status\t314.210306\t48.752777\t10.839700\t-0.194846\t-2.241042\t148.943145\t0.272000\t0.051000\n\t\n15:31:11.4\tlog_raw\tgps_raw\t#DUALANTENNAHEADINGA,USB3,0,48.0,FINESTEERING,2107,282689.400,02000000,d426,15824;INSUFFICIENT_OBS,NONE,-1.000000000,0.000000000,0.000000000,0.0,0.000000000,0.000000000,\"631T\",16,3,3,3,04,00,20,00*5af887b4\n\tsystem status\tnormal 2 28.000000 0 0\trobot status\t314.095782\t48.839969\t10.834000\t0.056755\t-2.354276\t149.149560\t0.369000\t-0.106000\n\t\n15:31:11.9\tlog_raw\tgps_raw\t#DUALANTENNAHEADINGA,USB3,0,48.0,FINESTEERING,2107,282689.900,02000000,d426,15824;INSUFFICIENT_OBS,NONE,-1.000000000,0.000000000,0.000000000,0.0,0.000000000,0.000000000,\"631T\",14,3,3,3,04,00,20,00*97b3bf20\n\tsystem status\tnormal 2 28.000000 0 0\trobot status\t313.981792\t48.926873\t10.827200\t0.255320\t-2.405738\t149.258946\t0.339000\t-0.063000\n\t\n15:31:12.4\tlog_raw\tgps_raw\t#DUALANTENNAHEADINGA,USB3,0,52.0,FINESTEERING,2107,282690.400,02000000,d426,15824;INSUFFICIENT_OBS,NONE,-1.000000000,0.000000000,0.000000000,0.0,0.000000000,0.000000000,\"631T\",13,3,3,3,04,00,20,00*a378a124\n\tsystem status\tnormal 2 28.000000 0 0\trobot status\t313.869462\t49.009955\t10.820700\t0.251213\t-2.160193\t149.316448\t0.328000\t-0.045000\n\t\n15:31:12.9\tlog_raw\tgps_raw\t#DUALANTENNAHEADINGA,USB3,0,52.0,FINESTEERING,2107,282690.900,02000000,d426,15824;INSUFFICIENT_OBS,NONE,-1.000000000,0.000000000,0.000000000,0.0,0.000000000,0.000000000,\"631T\",14,3,3,3,04,00,20,00*50b9140a\n\tsystem status\tnormal 2 28.000000 0 0\trobot status\t313.756339\t49.093291\t10.812900\t0.257274\t-1.971750\t149.387965\t0.320000\t-0.029000\n\t\n15:31:13.4\tlog_raw\tgps_raw\t#DUALANTENNAHEADINGA,USB3,0,51.5,FINESTEERING,2107,282691.400,02000000,d426,15824;INSUFFICIENT_OBS,NONE,-1.000000000,0.000000000,0.000000000,0.0,0.000000000,0.000000000,\"631T\",16,3,3,3,04,00,20,00*099db567\n\tsystem status\tnormal 2 28.000000 0 0\trobot status\t313.641315\t49.177615\t10.805100\t0.278679\t-1.927239\t149.463838\t0.340000\t-0.067000\n\t\n15:31:13.9\tlog_raw\tgps_raw\t#DUALANTENNAHEADINGA,USB3,0,51.5,FINESTEERING,2107,282691.900,02000000,d426,15824;INSUFFICIENT_OBS,NONE,-1.000000000,0.000000000,0.000000000,0.0,0.000000000,0.000000000,\"631T\",16,3,3,3,04,00,20,00*b0628b02\n\tsystem status\tnormal 2 28.000000 0 0\trobot status\t313.525004\t49.263420\t10.796800\t0.389125\t-1.831793\t149.475318\t0.270000\t0.032000\n\t\n15:31:14.4\tlog_raw\tgps_raw\t#DUALANTENNAHEADINGA,USB3,0,50.5,FINESTEERING,2107,282692.400,02000000,d426,15824;INSUFFICIENT_OBS,NONE,-1.000000000,0.000000000,0.000000000,0.0,0.000000000,0.000000000,\"631T\",16,3,3,3,04,00,20,00*dbb16ea8\n\tsystem status\tnormal 2 28.000000 0 0\trobot status\t313.412037\t49.346083\t10.792000\t0.347567\t-1.782122\t149.516505\t0.375000\t-0.104000\n\t\n15:31:14.9\tlog_raw\tgps_raw\t#DUALANTENNAHEADINGA,USB3,0,50.5,FINESTEERING,2107,282692.900,02000000,d426,15824;INSUFFICIENT_OBS,NONE,-1.000000000,0.000000000,0.000000000,0.0,0.000000000,0.000000000,\"631T\",16,3,3,3,04,00,20,00*624e50cd\n\tsystem status\tnormal 2 28.000000 0 0\trobot status\t313.295615\t49.431177\t10.788400\t0.343769\t-1.939218\t149.538955\t0.252000\t0.066000\n\t\n15:31:15.4\tlog_raw\tgps_raw\t#DUALANTENNAHEADINGA,USB3,0,49.5,FINESTEERING,2107,282693.400,02000000,d426,15824;INSUFFICIENT_OBS,NONE,-1.000000000,0.000000000,0.000000000,0.0,0.000000000,0.000000000,\"631T\",16,3,3,3,04,00,20,00*97362650\n\tsystem status\tnormal 2 28.000000 0 0\trobot status\t313.177682\t49.515812\t10.782800\t0.293010\t-2.019929\t149.497501\t0.269000\t0.031000\n\t\n15:31:15.9\tlog_raw\tgps_raw\t\tsystem status\tnormal 2 28.000000 0 0\trobot status\t313.062797\t49.598548\t10.777500\t0.161554\t-1.970979\t149.412622\t0.274000\t0.032000\n\t\n15:31:16.4\tlog_raw\tgps_raw\t#DUALANTENNAHEADINGA,USB3,0,49.5,FINESTEERING,2107,282694.400,02000000,d426,15824;INSUFFICIENT_OBS,NONE,-1.000000000,0.000000000,0.000000000,0.0,0.000000000,0.000000000,\"631T\",16,3,3,3,04,00,20,00*4d4f3e1e\n\tsystem status\tnormal 2 28.000000 0 0\trobot status\t312.949432\t49.682091\t10.772500\t0.147449\t-1.904516\t149.380629\t0.346000\t-0.072000\n\t\n15:31:16.9\tlog_raw\tgps_raw\t#DUALANTENNAHEADINGA,USB3,0,49.5,FINESTEERING,2107,282694.900,02000000,d426,15824;INSUFFICIENT_OBS,NONE,-1.000000000,0.000000000,0.000000000,0.0,0.000000000,0.000000000,\"631T\",16,3,3,3,04,00,20,00*f4b0007b\n\tsystem status\tnormal 2 28.000000 0 0\trobot status\t312.834563\t49.767879\t10.766500\t0.115880\t-1.908539\t149.275769\t0.342000\t-0.082000\n\t\n15:31:17.4\tlog_raw\tgps_raw\t#DUALANTENNAHEADINGA,USB3,0,47.5,FINESTEERING,2107,282695.400,02000000,d426,15824;INSUFFICIENT_OBS,NONE,-1.000000000,0.000000000,0.000000000,0.0,0.000000000,0.000000000,\"631T\",15,3,3,3,04,00,20,00*95eef455\n\tsystem status\tnormal 2 28.000000 0 0\trobot status\t312.718841\t49.853194\t10.760900\t0.084062\t-1.816787\t149.177172\t0.309000\t-0.019000\n\t\n15:31:17.9\tlog_raw\tgps_raw\t#DUALANTENNAHEADINGA,USB3,0,47.5,FINESTEERING,2107,282695.900,02000000,d426,15824;INSUFFICIENT_OBS,NONE,-1.000000000,0.000000000,0.000000000,0.0,0.000000000,0.000000000,\"631T\",15,3,3,3,04,00,20,00*2c11ca30\n\tsystem status\tnormal 2 28.000000 0 0\trobot status\t312.605645\t49.937179\t10.755600\t-0.001097\t-1.818552\t149.084094\t0.294000\t0.001000\n\t\n15:31:18.4\tlog_raw\tgps_raw\t#DUALANTENNAHEADINGA,USB3,0,48.0,FINESTEERING,2107,282696.400,02000000,d426,15824;INSUFFICIENT_OBS,NONE,-1.000000000,0.000000000,0.000000000,0.0,0.000000000,0.000000000,\"631T\",15,3,3,3,04,00,20,00*0497816d\n\tsystem status\tnormal 2 28.000000 0 0\trobot status\t312.494808\t50.020200\t10.751600\t-0.016721\t-1.847811\t148.986730\t0.304000\t-0.006000\n\t\n15:31:18.9\tlog_raw\tgps_raw\t#DUALANTENNAHEADINGA,USB3,0,48.0,FINESTEERING,2107,282696.900,02000000,d426,15824;INSUFFICIENT_OBS,NONE,-1.000000000,0.000000000,0.000000000,0.0,0.000000000,0.000000000,\"631T\",16,3,3,3,04,00,20,00*1e3e39a1\n\tsystem status\tnormal 2 28.000000 0 0\trobot status\t312.378487\t50.107723\t10.746200\t0.019321\t-1.953920\t148.834172\t0.307000\t-0.013000\n\t\n15:31:19.4\tlog_raw\tgps_raw\t\tsystem status\tnormal 2 28.000000 0 0\trobot status\t312.269615\t50.190791\t10.742300\t-0.027098\t-1.964723\t148.759448\t0.311000\t-0.013000\n\t\n15:31:19.9\tlog_raw\tgps_raw\t#DUALANTENNAHEADINGA,USB3,0,47.0,FINESTEERING,2107,282697.900,02000000,d426,15824;INSUFFICIENT_OBS,NONE,-1.000000000,0.000000000,0.000000000,0.0,0.000000000,0.000000000,\"631T\",18,3,3,3,04,00,20,00*95f0b571\n\tsystem status\tnormal 2 28.000000
